vi "ReadWait.vi"(6 "Numeric":dbl, 8 "error in (no error)":errorcluster, 9 "Value":bool=TRUE, 10 "Read":i32, 11 "I-O in":refnum<class "I-O.lvclass">) -> (0 "error out":errorcluster, 3 "I-O out":refnum<class "I-O.lvclass">)   [LabVIEW 2021, in "I-O.lvclass"]
uses:
  I-O.lvclass
  <vilib>/Utility/file.llb/Read Delimited Spreadsheet (string).vi
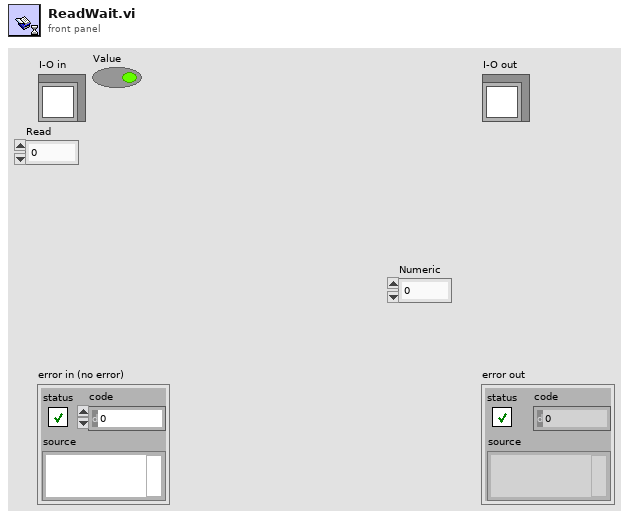
[diagram p1: front panel]
types:
  T1 = typedef "File Paths.ctl" = cluster{"Glue Pattern Folder":path, "Carrier Tray Folder":path, "Pick Up Tool Fixture Folder":path, "Components Folder":path, "Bellows Tool Offset.txt":path, "Pick Up Tool Offset.txt":path, "Dispense Tip Offset.txt":path, "Log Files":path, "Gantry Assembly Map.txt":path, "Syringe and offset map.txt":path, "Controllers Folder":path, "Local dbase config":path}
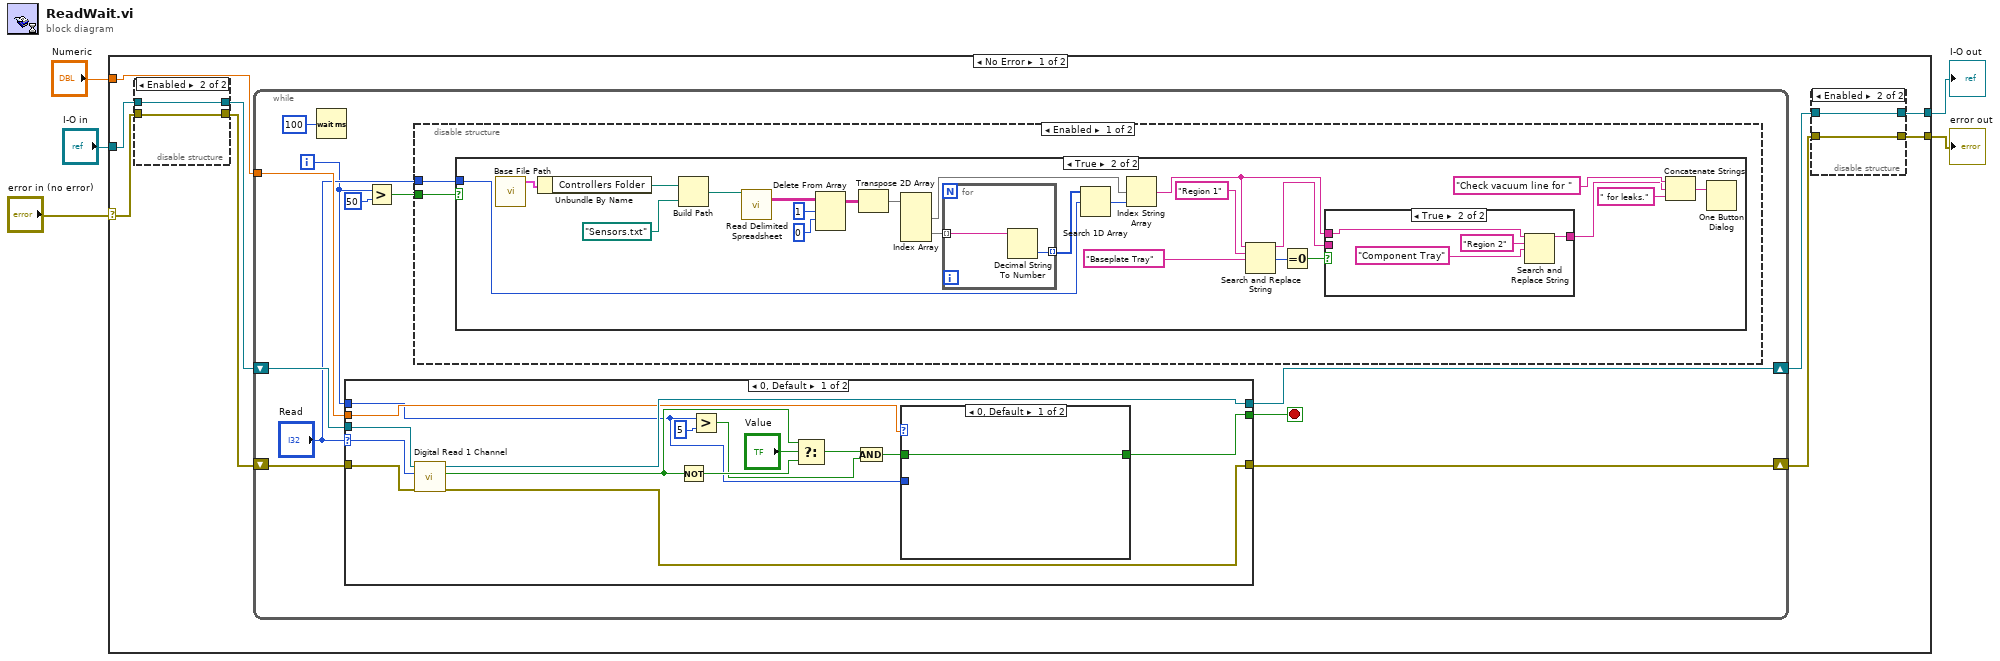
[diagram p0: block diagram]
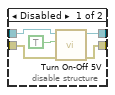
[diagram p2: hidden frame]
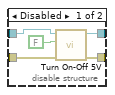
[diagram p3: hidden frame]
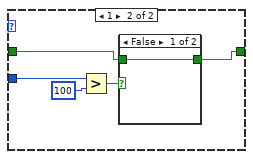
[diagram p7: hidden frame]
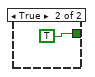
[diagram p8: hidden frame]
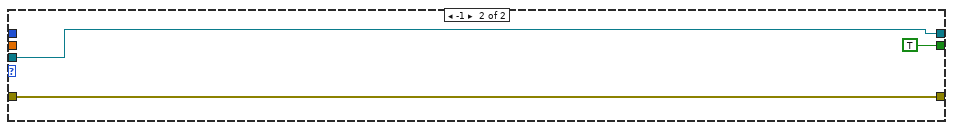
[diagram p9: hidden frame]
diagram:
  n1 = case shown="No Error" "error in (no error)" {
    selector: "error in (no error)" -> [w10 w100]
    tunnel: [w7 w100] -> w4
    tunnel: [w13 w99] -> w2
    tunnel: "I-O in" -> [w14 w99]
    tunnel: "Numeric" -> [w6 _]
    frame No Error {
      n2 = disable-structure shown="Enabled" {
        disable-tunnel: w14 -> [w19 w21]
        disable-tunnel: [w18 w21] -> w12
        disable-tunnel: w10 -> [w17 w20]
        disable-tunnel: [w16 w20] -> w9
        frame Disabled {
          n3 = call-dynamic "Turn On-Off 5V.vi"("error in (no error)"=w17, "Value"=TRUE, "I-O in"=w19) -> ("error out"=w16:errorcluster, "I-O out"=w18:refnum<class "I-O.lvclass">)  [unwired: 7 in]
        }
        frame Enabled {
        }
      }
      n4 = while {
        shift-right: [w37] -> w11
        shift-left: w12 -> [w33]
        shift-right: [w35] -> w8
        shift-left: w9 -> [w36]
        tunnel: w6 -> [w34]
        i -> [w31]
        stop <- w38 stop-if-true
        n5 = Wait (ms)(milliseconds to wait=u32 100) -> ()  [unwired: 1 out]
        n6 = case shown="0, Default" "Read" {
          selector: "Read" -> [w79 _]
          tunnel: w31 -> [w73 _]
          tunnel: [w76 TRUE] -> w38
          tunnel: w33 -> [w83 w98]
          tunnel: [w82 w98] -> w37
          tunnel: w36 -> [w81 w96]
          tunnel: [w80 w96] -> w35
          tunnel: w34 -> [w74 _]
          frame 0, Default {
            n7 = call-dynamic "Digital Read 1 Channel.vi"("error in (no error)"=w81, "Read"=w79, "I-O in"=w83) -> ("error out"=w80:errorcluster, "Value"=w77:bool, "I-O out"=w82:refnum<class "I-O.lvclass">)  [unwired: 6 in]
            n8 = Not(x=w77) -> (.not. x?=w87:bool)
            n9 = Greater?(x=w73, y=5) -> (0:w84:bool)
            n10 = Select(t=w77, s="Value", f=w87) -> (s? t:f=w85:bool)
            n11 = And(x=w85, y=w84) -> (x .and. y?=w75:bool)
            n12 = case shown="0, Default" w74 {
              tunnel: [w88 w93] -> w76
              tunnel: w75 -> [w88 w92]
              tunnel: w73 -> [_ w91]
              frame 0, Default {
              }
              frame 1 {
                n13 = Greater?(x=w91, y=100) -> (0:w90:bool)
                n14 = case shown="False" w90 {
                  tunnel: [w94 TRUE] -> w93
                  tunnel: w92 -> [w94 _]
                  frame False {
                  }
                  frame True {
                  }
                }
              }
            }
          }
          frame -1 {
          }
        }
        n15 = Greater?(x=w31, y=50) -> (0:w29:bool)
        n16 = disable-structure shown="Enabled" {
          disable-tunnel: "Read" -> [w41 _]
          disable-tunnel: w29 -> [w40 _]
          frame Enabled {
            n17 = case shown="True" w40 {
              tunnel: w41 -> [_ w65]
              frame False {
              }
              frame True {
                n18 = call "Base File Path.vi"() -> ("Paths Out"=w64:T1)  [unwired: 11 in]
                n19 = Unbundle By Name(w64) -> ("Controllers Folder"=w63:path)
                n20 = Build Path(base path=w63, name or relative path=path "Sensors.txt") -> (appended path=w61:path)
                n21 = call-poly <vilib>:"Read Delimited Spreadsheet.vi"("file path (dialog if empty)"=w61) -> ("all rows"=w60:string[][])  [unwired: 9 in, 5 out]
                n22 = Delete From Array(array=w60, length=1, index (row)=0) -> (array with subset deleted=w57:string[][])  [unwired: 1 in, 1 out]
                n23 = Transpose 2D Array(2D array=w57) -> (transposed array=w56:string[][])
                n24 = Index Array(array=w56) -> (element #1=w53:string[], element #2=w55:string[])  [unwired: 4 in]
                n25 = for {
                  tunnel: w55 -> [w72] mode=indexing
                  tunnel: [w71] -> w54 mode=indexing
                  n26 = Decimal String To Number(string=w72) -> (number=w71:i32)  [unwired: 2 in, 1 out]
                }
                n27 = Search 1D Array(1D array=w54, element=w65) -> (index of element=w52:i32)  [unwired: 1 in]
                n28 = Index String Array(1:w52, 2:w53) -> (0:w44:string)  [unwired: 1 in]
                n29 = Search and Replace String(input string=w44, search string="Region 1" ("replace string (\"\")"), replace string="Baseplate Tray" ("replace string (\"\")")) -> (result string=w42:string, number of replacements=w46:i32)  [unwired: 5 in, 2 out]
                n30 = Equal To 0?(x=w46) -> (x = 0?=w45:bool)
                n31 = case shown="True" w45 {
                  tunnel: w44 -> [_ w70]
                  tunnel: [w66 w67] -> w43
                  tunnel: w42 -> [w66 _]
                  frame False {
                  }
                  frame True {
                    n32 = Search and Replace String(input string=w70, search string="Region 2", replace string="Component Tray" ("replace string (\"\")")) -> (result string=w67:string)  [unwired: 5 in, 3 out]
                  }
                }
                n33 = Concatenate Strings("Check vacuum line for " ("message"), w43, " for leaks." ("string")) -> (w49:string)
                n34 = One Button Dialog(message=w49) -> ()  [unwired: 1 in, 1 out]
              }
            }
          }
          frame Disabled {
          }
        }
      }
      n35 = disable-structure shown="Enabled" {
        disable-tunnel: [w26 w28] -> w13
        disable-tunnel: w11 -> [w25 w28]
        disable-tunnel: w8 -> [w24 w27]
        disable-tunnel: [w23 w27] -> w7
        frame Disabled {
          n36 = call-dynamic "Turn On-Off 5V.vi"("error in (no error)"=w24, "Value"=FALSE, "I-O in"=w25) -> ("error out"=w23:errorcluster, "I-O out"=w26:refnum<class "I-O.lvclass">)  [unwired: 7 in]
        }
        frame Enabled {
        }
      }
    }
    frame Error {
    }
  }
  "error out" <- w4
  "I-O out" <- w2
